vi "GetData2.vi"() -> ()   [LabVIEW 2017]
uses:
  <vilib>/Utility/file.llb/Read Delimited Spreadsheet (string).vi
  <vilib>/Utility/file.llb/Write Delimited Spreadsheet (string).vi
panel:
  out "Numeric":i32
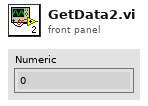
[diagram p1: front panel]
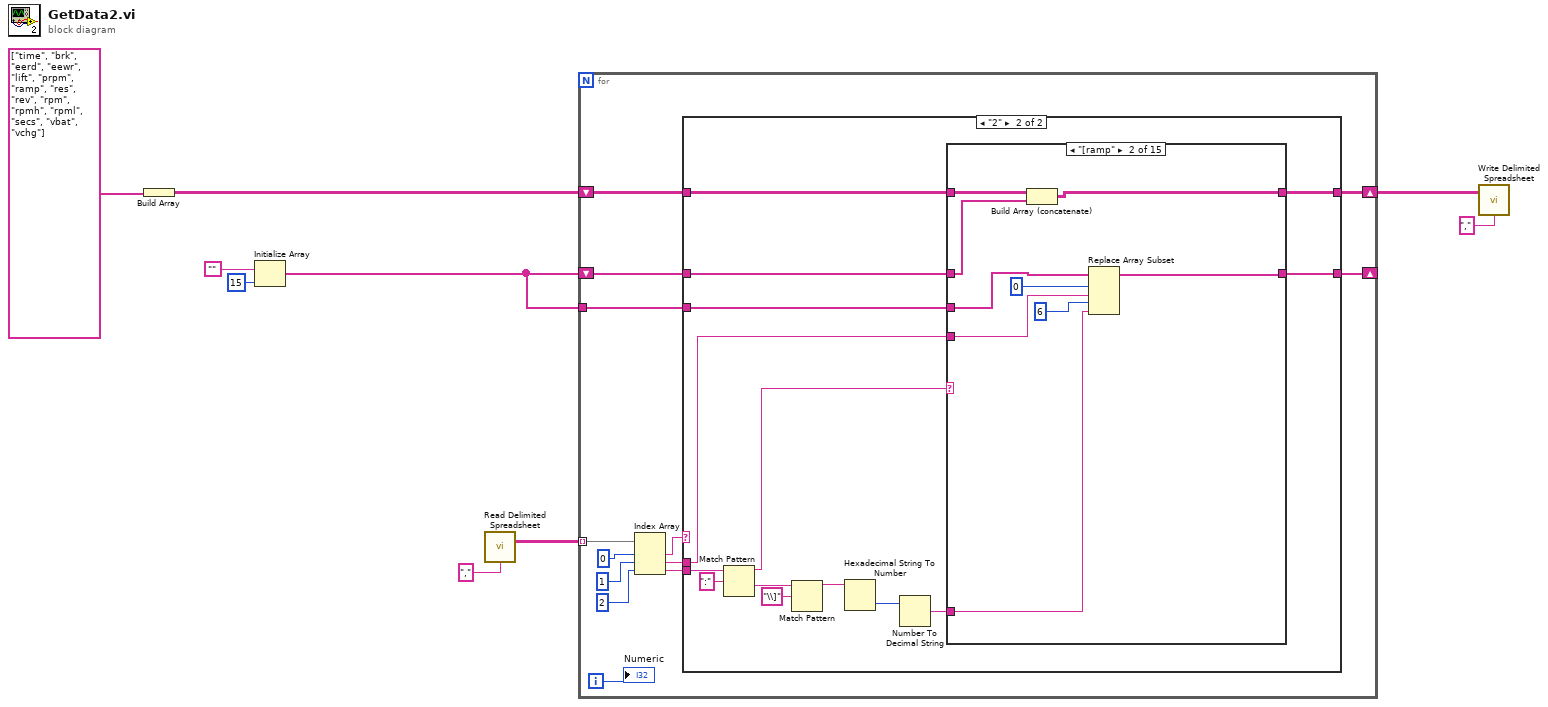
[diagram p0: block diagram]
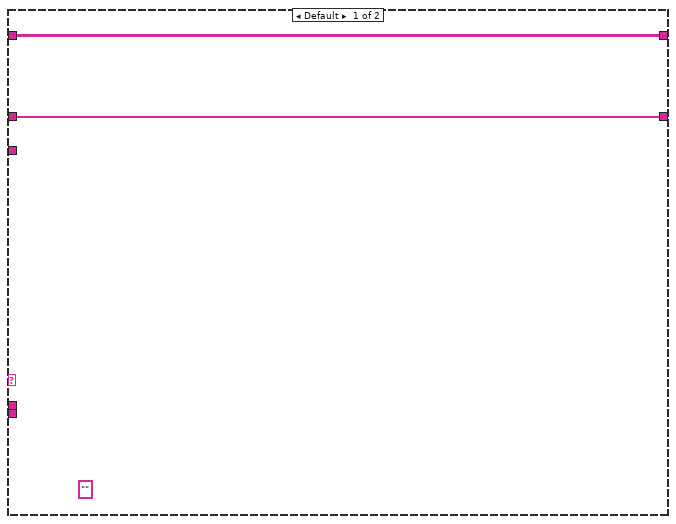
[diagram p2: hidden frame]
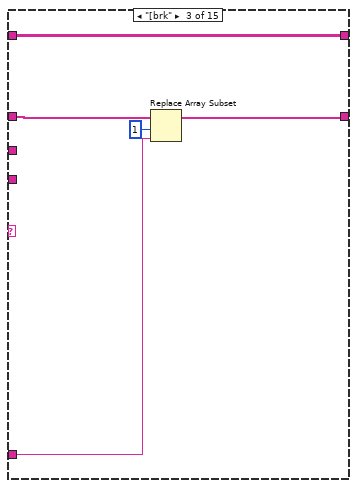
[diagram p4: hidden frame]
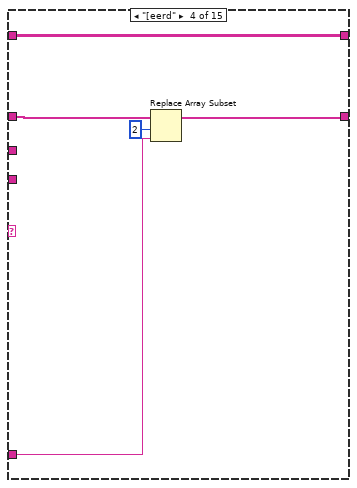
[diagram p5: hidden frame]
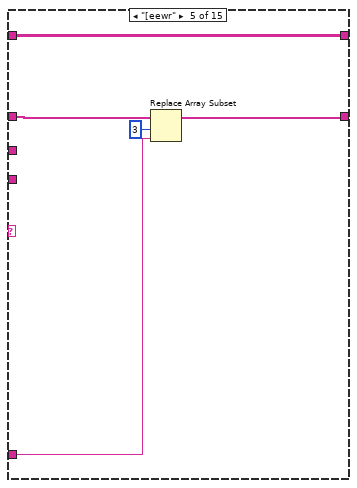
[diagram p6: hidden frame]
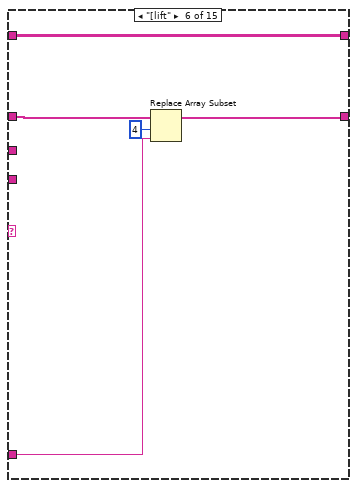
[diagram p7: hidden frame]
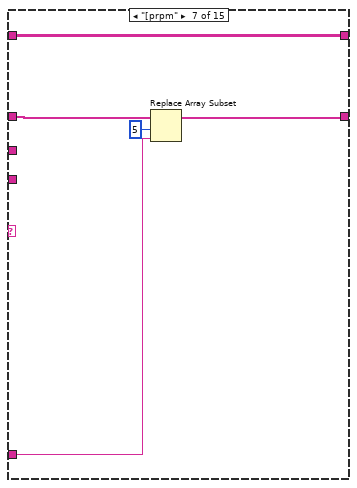
[diagram p8: hidden frame]
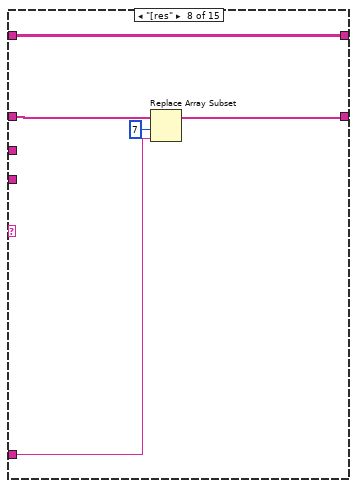
[diagram p9: hidden frame]
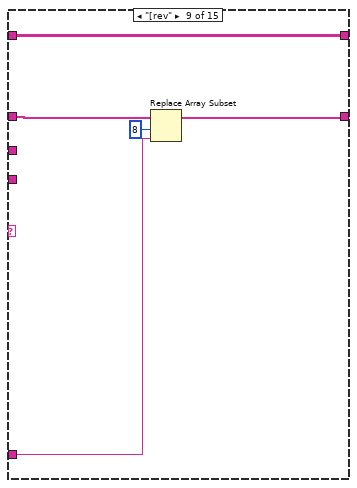
[diagram p10: hidden frame]
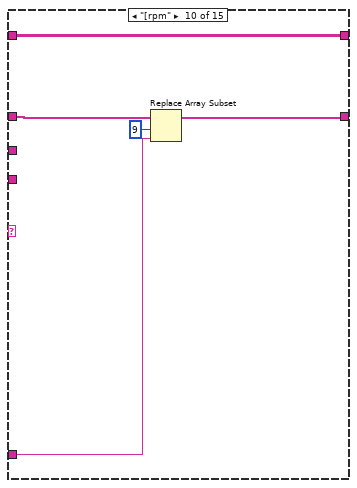
[diagram p11: hidden frame]
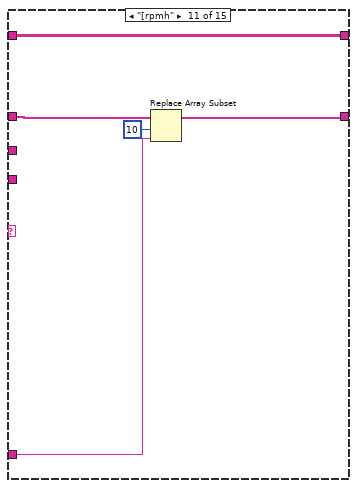
[diagram p12: hidden frame]
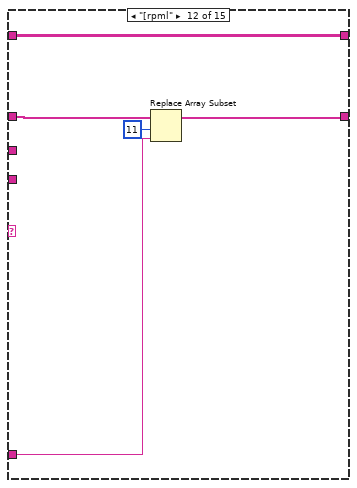
[diagram p13: hidden frame]
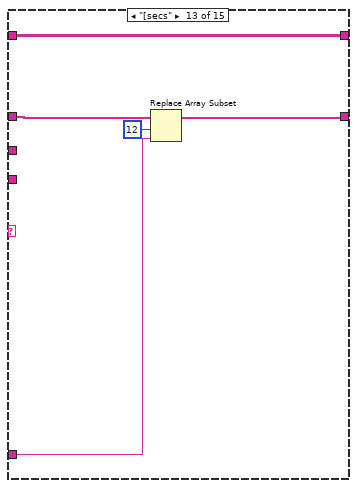
[diagram p14: hidden frame]
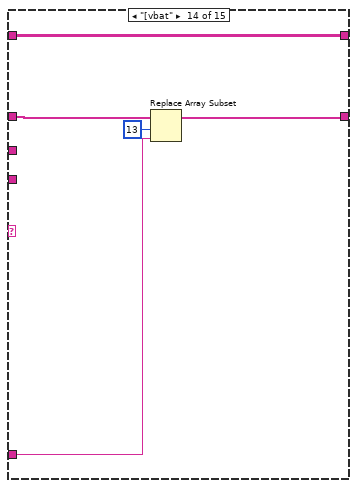
[diagram p15: hidden frame]
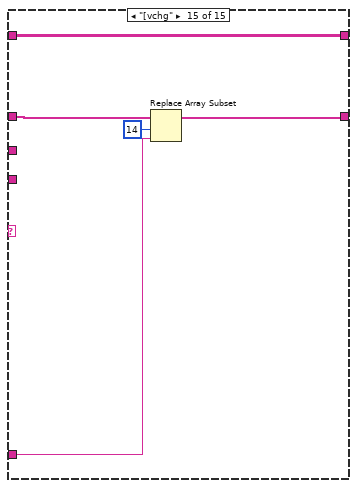
[diagram p16: hidden frame]
diagram:
  n1 = Build Array(string[] ["time", "brk", "eerd", "eewr", "lift", "prpm", "ramp", "res", "rev", "rpm", "rpmh", "rpml", "secs", "vbat", "vchg"]) -> (w7:string[][])
  n2 = Initialize Array("", 15 ("dimension size")) -> (w1:string[])
  n3 = call-poly <vilib>:"Read Delimited Spreadsheet.vi"("delimiter (\\t)"="," ("delimiter (\\t)")) -> ("all rows"=w9:string[][])  [unwired: 9 in, 5 out]
  n4 = for {
    tunnel: w9 -> [w22] mode=indexing
    shift-right: [w14] -> w4
    shift-left: w7 -> [w16]
    shift-right: [w13] -> _
    shift-left: w1 -> [w15]
    tunnel: w1 -> [w11]
    i -> [w10]
    n5 = Index Array(array=w22, index #1=0 ("index"), index #2=1 ("index"), index #3=2 ("index")) -> (element #1=w12:string, element #2=w18:string, element #3=w17:string)
    n6 = case shown="\"2\"" w12 {
      tunnel: w18 -> [_ w27]
      tunnel: w17 -> [_ w38]
      tunnel: w16 -> [w24 w30]
      tunnel: w15 -> [w23 w28]
      tunnel: [w24 w31] -> w14
      tunnel: [w23 w29] -> w13
      tunnel: w11 -> [_ w25]
      frame Default {
        (unwired) "" ("String")
      }
      frame "2" {
        n7 = Match Pattern(string=w38, regular expression=":") -> (before substring=w26:string, after substring=w36:string)  [unwired: 1 in, 2 out]
        n8 = Match Pattern(string=w36, regular expression="\\]") -> (before substring=w34:string)  [unwired: 1 in, 3 out]
        n9 = Hexadecimal String To Number(string=w34) -> (number=w33:u32)  [unwired: 2 in, 1 out]
        n10 = Number To Decimal String(number=w33) -> (decimal integer string=w32:string)  [unwired: 1 in]
        n11 = case shown="\"[ramp\"" w26 {
          tunnel: w32 -> [_ w43 w51 w56 w61 w66 w71 w76 w81 w86 w91 w96 w101 w106 w111]
          tunnel: [w40 w48 w52 w57 w62 w67 w72 w77 w82 w87 w92 w97 w102 w107 w112] -> w31
          tunnel: w30 -> [w40 w49 w52 w57 w62 w67 w72 w77 w82 w87 w92 w97 w102 w107 w112]
          tunnel: [w39 w42 w53 w58 w63 w68 w73 w78 w83 w88 w93 w98 w103 w108 w113] -> w29
          tunnel: w28 -> [w39 w47 w54 w59 w64 w69 w74 w79 w84 w89 w94 w99 w104 w109 w114]
          tunnel: w27 -> [_ w45 _ _ _ _ _ _ _ _ _ _ _ _ _]
          tunnel: w25 -> [_ w41 _ _ _ _ _ _ _ _ _ _ _ _ _]
          frame Default {
          }
          frame "[ramp" {
            n12 = Build Array (concatenate)(w49, w47) -> (w48:string[][])
            n13 = Replace Array Subset(array=w41, new element #1=w45, index #1=0 ("index"), new element #2=w43, index #2=6 ("index")) -> (w42:string[])
          }
          frame "[brk" {
            n14 = Replace Array Subset(array=w54, new element=w51, index=1) -> (w53:string[])
          }
          frame "[eerd" {
            n15 = Replace Array Subset(array=w59, new element=w56, index=2) -> (w58:string[])
          }
          frame "[eewr" {
            n16 = Replace Array Subset(array=w64, new element=w61, index=3) -> (w63:string[])
          }
          frame "[lift" {
            n17 = Replace Array Subset(array=w69, new element=w66, index=4) -> (w68:string[])
          }
          frame "[prpm" {
            n18 = Replace Array Subset(array=w74, new element=w71, index=5) -> (w73:string[])
          }
          frame "[res" {
            n19 = Replace Array Subset(array=w79, new element=w76, index=7) -> (w78:string[])
          }
          frame "[rev" {
            n20 = Replace Array Subset(array=w84, new element=w81, index=8) -> (w83:string[])
          }
          frame "[rpm" {
            n21 = Replace Array Subset(array=w89, new element=w86, index=9) -> (w88:string[])
          }
          frame "[rpmh" {
            n22 = Replace Array Subset(array=w94, new element=w91, index=10) -> (w93:string[])
          }
          frame "[rpml" {
            n23 = Replace Array Subset(array=w99, new element=w96, index=11) -> (w98:string[])
          }
          frame "[secs" {
            n24 = Replace Array Subset(array=w104, new element=w101, index=12) -> (w103:string[])
          }
          frame "[vbat" {
            n25 = Replace Array Subset(array=w109, new element=w106, index=13) -> (w108:string[])
          }
          frame "[vchg" {
            n26 = Replace Array Subset(array=w114, new element=w111, index=14) -> (w113:string[])
          }
        }
      }
    }
    "Numeric" <- w10
  }
  n27 = call-poly <vilib>:"Write Delimited Spreadsheet.vi"("2D data"=w4, "delimiter (\\t)"="," ("delimiter (\\t)")) -> ()  [unwired: 12 in, 2 out]
